vi "DG535.SetDelay.vi"(0 "i ref in":refnum<vi>, 7 "A Delay":dbl min=0.0 max=999.999999999995 format="%.12f", 11 "error in (no error)":errorcluster) -> (4 "i ref out":refnum<vi>, 15 "error out":errorcluster)   [LabVIEW 2014, in "DG535.lvlib"]
uses:
  DG535.lvlib
panel:
  # "+"
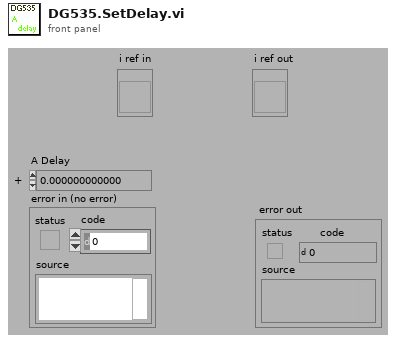
[diagram p1: front panel]
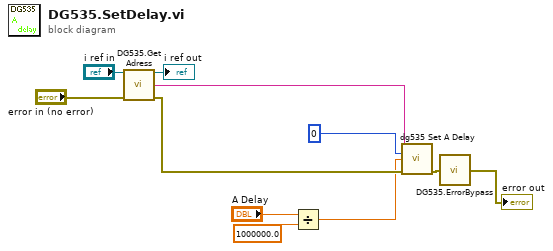
[diagram p0: block diagram]
diagram:
  n1 = call "DG535.Get Adress.vi"("i ref in"="i ref in", "error in (no error)"="error in (no error)") -> ("i ref out"=→"i ref out":refnum<vi>, "address"=w8:string, "error out"=w7:errorcluster)  [unwired: 10 in, 1 out]
  n2 = Divide(x="A Delay", y=1000000.0) -> (x/y=w2:dbl)
  n3 = call "dg535 Set A Delay.vi"("address string"=w8, "A="=0, "A"=w2, "error in"=w7) -> ("error out"=w6:errorcluster)  [unwired: 11 in]
  n4 = call "DG535.ErrorBypass.vi"("error in (no error)"=w6) -> ("error out"=→"error out":errorcluster)  [unwired: 14 in]
